vi "rename tag.vi"(8 "error in":errorcluster, 9 "new tag name":string, 10 "current tag name":string, 11 "tag collection in":refnum<class "data bus tag collection.lvclass">) -> (0 "error out":errorcluster, 3 "tag collection out":refnum<class "data bus tag collection.lvclass">)   [LabVIEW 2013, in "data bus tag collection.lvclass"]
uses:
  data bus tag collection.lvclass
  tag/data bus tag description.lvclass/data bus tag description.ctl
  tag/data bus tag description.lvclass
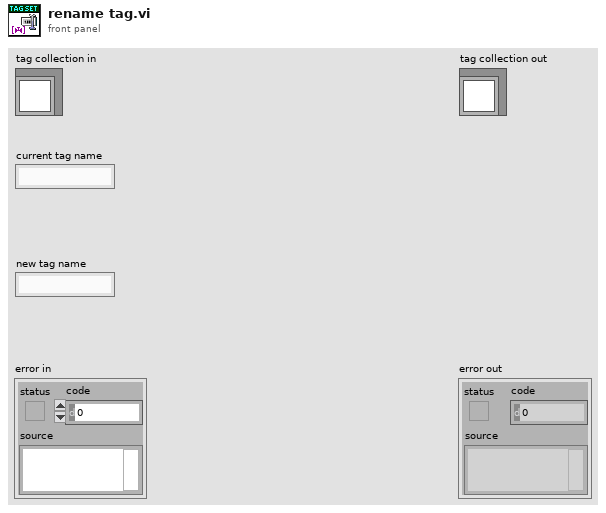
[diagram p1: front panel]
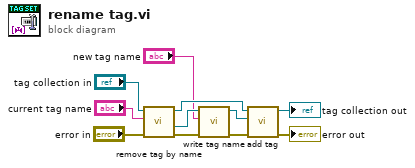
[diagram p0: block diagram]
diagram:
  n1 = call "remove tag by name.vi"("error in"="error in", "tag"="current tag name", "tag collection in"="tag collection in") -> ("error out"=w9:errorcluster, "removed tag"=w8:refnum<class "data bus tag description.lvclass">, "tag collection out"=w4:refnum<class "data bus tag collection.lvclass">)  [unwired: 6 in]
  n2 = call "write tag name.vi"("error in"=w9, "name"="new tag name", "system tag in"=w8) -> ("error out"=w6:errorcluster, "system tag out"=w7:refnum<class "data bus tag description.lvclass">)  [unwired: 7 in]
  n3 = call "add tag.vi"("error in"=w6, "tag"=w7, "tag collection in"=w4) -> ("error out"=→"error out":errorcluster, "tag collection out"=→"tag collection out":refnum<class "data bus tag collection.lvclass">)  [unwired: 7 in]
